vi "Generate Waveform.vi"(8 "error in":errorcluster, 11 "Generator in":refnum<class "Generador.lvclass">) -> (0 "error out":errorcluster, 2 "Waveform":waveform(dbl), 3 "Generator out":refnum<class "Generador.lvclass">)   [LabVIEW 2020, in "FGen.lvlib" / "Generador.lvclass"]
uses:
  Generador.lvclass
  Generador.lvclass/Generador.ctl
  Get offset.vi
  Get signal type.vi
  Get frequency.vi
  Get amplitude.vi
  Get phase.vi
  Get sampling info.vi
  Get square wave duty cycle (%).vi
  <vilib>/measure/NI_MABase.lvlib
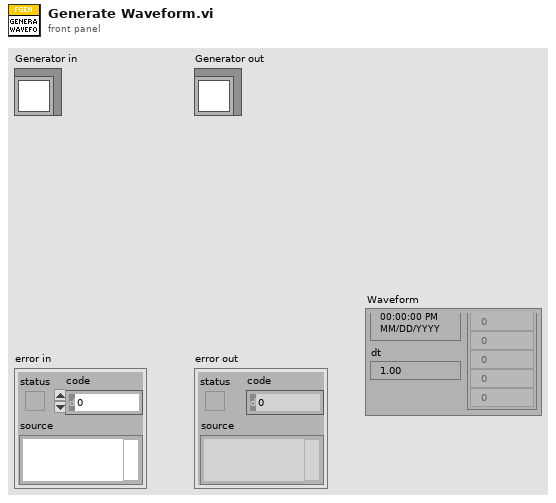
[diagram p1: front panel]
types:
  T1 = enum16{"Sine Wave", "Triangle Wave", "Square Wave", "Sawtooth Wave"}
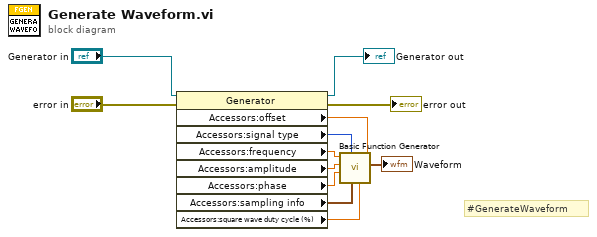
[diagram p0: block diagram]
diagram:
  # "#GenerateWaveform"
  n1 = property class="Generator"(reference="Generator in", error in="error in") -> (reference out=→"Generator out":refnum<class "Generador.lvclass">, error out=→"error out":errorcluster, "Accessors:offset"=w9:dbl, "Accessors:signal type"=w8:T1, "Accessors:frequency"=w7:dbl, "Accessors:amplitude"=w6:dbl, "Accessors:phase"=w5:dbl, "Accessors:sampling info"=w4:cluster{"Fs":dbl, "#s":dbl}, "Accessors:square wave duty cycle (%)"=w3:dbl)
  n2 = call <vilib>:"Basic Function Generator.vi"("offset"=w9, "square wave duty cycle (%)"=w3, "sampling info"=w4, "signal type"=w8, "phase"=w5, "amplitude"=w6, "frequency"=w7) -> ("signal out"=→"Waveform":waveform(dbl))  [unwired: 2 in, 2 out]
